vi "Write SuBUS.vi"(5 "sample rate":dbl=20000000.0 format="%#_13p", 7 "OVS":u8=16, 8 "Error In":errorcluster, 9 "Reg_Address_Data":T2={"Address"=81, "Data"=0} {"Address" format="%.0x"}, 10 "USID":T1=13 max=15, 11 "HSDIO Sessions":T3) -> (0 "Error Out":errorcluster)   [LabVIEW 2013]
uses:
  Controls/Reg_Address_Data.ctl
  Controls/USID.ctl
  <instrlib>/niHSDIO/niHSDIO.llb/niHSDIO Write Named Waveform (WDT).vi
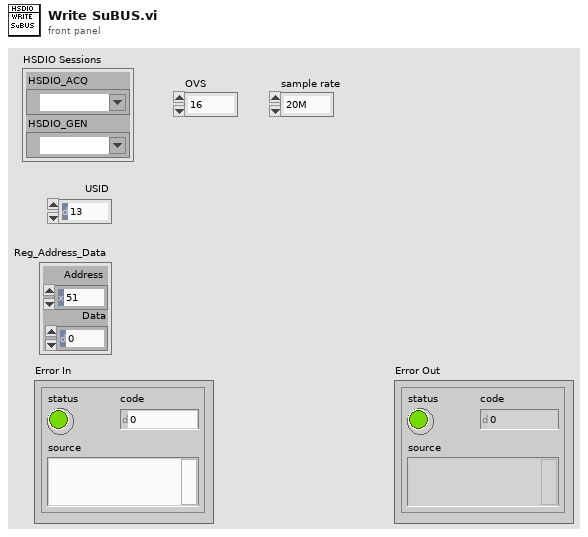
[diagram p1: front panel]
types:
  T1 = typedef "USID.ctl" = u8
  T2 = typedef "Reg_Address_Data.ctl" = cluster{"Address":u8, "Data":u8}
  T3 = cluster{"HSDIO_ACQ":refnum<k15>, "HSDIO_GEN":refnum<k15>}
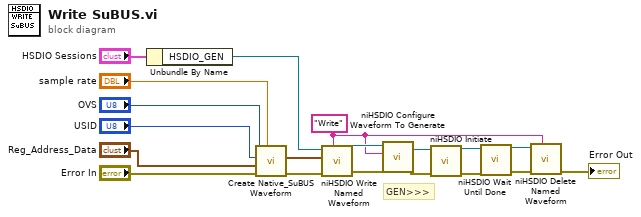
[diagram p0: block diagram]
diagram:
  w10 = "Write" ("waveform name (default:\"\")")
  # "GEN>>>"
  n1 = Unbundle By Name("HSDIO Sessions") -> ("HSDIO_GEN"=w7:refnum<k15>)
  n2 = call "Create Native_SuBUS Waveform.vi"("sample rate"="sample rate", "error in (no error)"="Error In", "Reg_Address_Data"="Reg_Address_Data", "USID"="USID", "OVS"="OVS") -> ("error out"=w9:errorcluster, "Digital Waveform Graph"=w8:digitalwaveform)  [unwired: 5 in]
  n3 = call-poly <instrlib>:"niHSDIO Write Named Waveform.vi"("waveform name (default:\"\")"=w10, "error in (no error)"=w9, "data"=w8, "instrument handle"=w7) -> ("error out"=w16:errorcluster, "instrument handle out"=w15:refnum<k15>)  [unwired: 6 in]
  n4 = call <instrlib>:"niHSDIO Configure Waveform To Generate.vi"("error in (no error)"=w16, "waveform name"=w10, "instrument handle"=w15) -> ("error out"=w13:errorcluster, "instrument handle out"=w14:refnum<k15>)  [unwired: 7 in]
  n5 = call <instrlib>:"niHSDIO Initiate.vi"("error in (no error)"=w13, "instrument handle"=w14) -> ("error out"=w18:errorcluster, "instrument handle out"=w17:refnum<k15>)  [unwired: 8 in]
  n6 = call <instrlib>:"niHSDIO Wait Until Done.vi"("error in (no error)"=w18, "instrument handle"=w17) -> ("error out"=w12:errorcluster, "instrument handle out"=w11:refnum<k15>)  [unwired: 8 in]
  n7 = call <instrlib>:"niHSDIO Delete Named Waveform.vi"("waveform name (default:\"\")"=w10, "error in (no error)"=w12, "instrument handle"=w11) -> ("error out"=→"Error Out":errorcluster)  [unwired: 7 in, 1 out]
